vi "Get Identifier.vi"(8 "error in (no error)":errorcluster, 11 "NI-XNET CAN Writer Execution Unit in":refnum<class "NI-XNET CAN Writer Execution Unit.lvclass">) -> (0 "error out":errorcluster, 2 "Identifier":string, 3 "NI-XNET CAN Writer Execution Unit out":refnum<class "NI-XNET CAN Writer Execution Unit.lvclass">)   [LabVIEW 2020, in "Communication Bus Template Engine.lvlib" / "Implementation.lvlib" / "NI-XNET CAN Writer Execution Unit.lvclass"]
uses:
  NI-XNET CAN Writer Execution Unit.lvclass
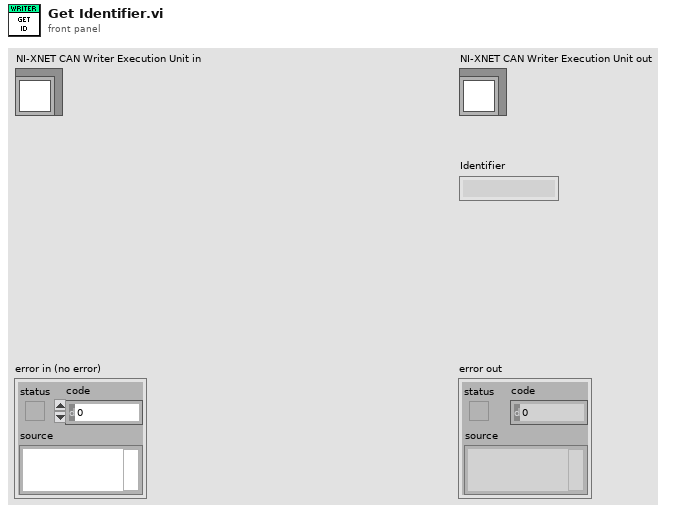
[diagram p1: front panel]
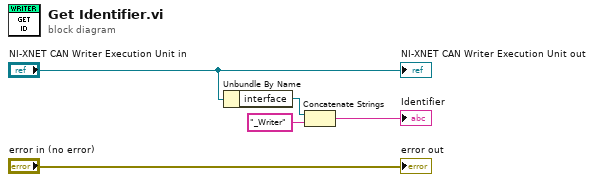
[diagram p0: block diagram]
diagram:
  n1 = Unbundle By Name("NI-XNET CAN Writer Execution Unit in") -> ("interface"=w4:refnum<k21>)
  n2 = Concatenate Strings(w4, "_Writer" ("string")) -> (→"Identifier":string)
  "error out" <- "error in (no error)"
  "NI-XNET CAN Writer Execution Unit out" <- "NI-XNET CAN Writer Execution Unit in"
